vi "Launch Instruments.vi"(8 "error in":errorcluster, 11 "Controller in":refnum<class "Controller.lvclass">) -> (0 "error out":errorcluster, 3 "Controller out":refnum<class "Controller.lvclass">)   [LabVIEW 2018, in "Controller.lvlib" / "Controller.lvclass"]
doc: "Configure the Instrument objects for operation and stuff them in their appropriate Instr Actor objects, calling their Pre Launch Init methods. The queues for these will be stored in the FGV for communication with the UI."
uses:
  Controller.lvclass
  PAS/Instrument/ePAS.lvclass
  C:/Users/Labview/Documents/exscalabar_server/reusable/Instrument/Instrument.lvclass
  CRDS/Main/eCRDS.lvclass
  reusable/PAS/Data/Main/PAS Data.lvclass
  C:/Users/Labview/Documents/exscalabar_server/reusable/Data/Data.lvclass
  Instr Actor/Instr Actor.lvclass
  C:/Users/Labview/Documents/exscalabar_server/SuperActor/SuperActor.lvclass
  C:/Program Files (x86)/National Instruments/LabVIEW 2018/vi.lib/ActorFramework/Actor/Actor.lvclass
  PAS/Data/Cell/ePAS Cell Data.lvclass
  C:/Users/Labview/Documents/exscalabar_server/reusable/PAS/Data/Cell/PAS Cell Data.lvclass
  Update Controller Data MSG.lvclass
  C:/Users/Labview/Documents/exscalabar_server/reusable/DAQ Device/Device/Generic Data Update Data MSG/Generic Update Data Message.lvclass
  reusable/Instrument/Instrument.lvclass/Instrument.ctl
  reusable/DAQ Device/Device/Generic Data Update Data MSG/Generic Update Data Message.lvclass/Generic Update Data Message.ctl
  Instr Actor/Instr Actor.lvclass/Instr Actor.ctl
  SuperActor/SuperActor.lvclass/SuperActor.ctl
  reusable/DAQ Device/Device/Generic Data Update Data MSG/Write ID.vi
  Instr Actor/Accessors/Write Instr.vi
  SuperActor/Write ID.vi
  Instr Actor/Accessors/Write Update Data MSG.vi
  reusable/Instrument/Write Data.vi
  reusable/PAS/Data/Main/Write CellData.vi
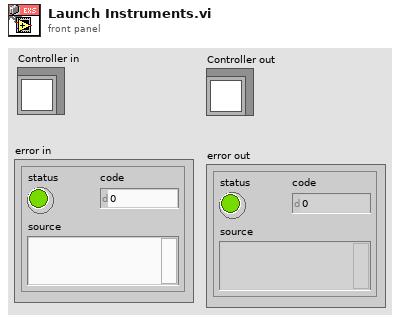
[diagram p1: front panel]
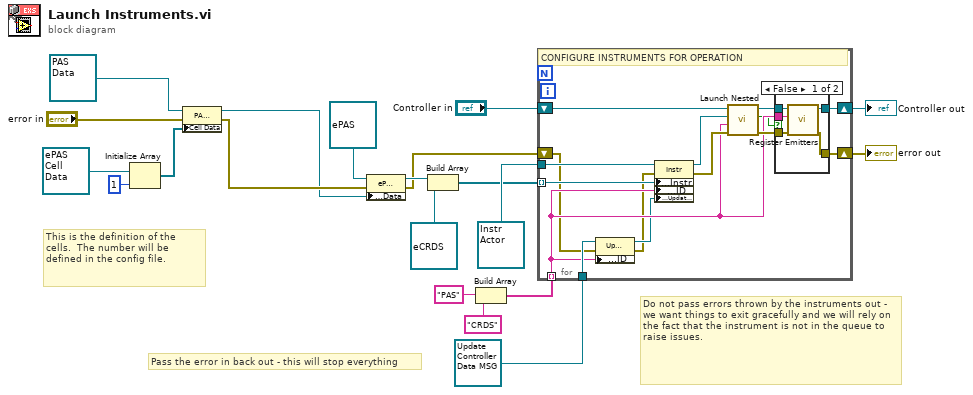
[diagram p0: block diagram]
diagram:
  # "This is the definition of the cells.  The number will be defined in the config file."
  # "Do not pass errors thrown by the instruments out - we want things to exit gracefully and we will rely on the fact that the instrument is not in the queue to raise issues."
  # "Pass the error in back out - this will stop everything"
  n1 = Initialize Array(refnum<class "ePAS Cell Data.lvclass"> refnum ("ePAS Cell"), 1 ("dimension size")) -> (w17:refnum<class "ePAS Cell Data.lvclass">[])
  n2 = property class="PAS Data"(reference=refnum<class "PAS Data.lvclass"> refnum ("PAS Data"), error in="error in", "Cell Data"=w17) -> (reference out=w11:refnum<class "PAS Data.lvclass">, error out=w18:errorcluster)
  n3 = property class="ePAS"(reference=refnum<class "ePAS.lvclass"> refnum ("ePAS.lvclass"), error in=w18, "Accessors:Data"=w11) -> (reference out=w15:refnum<class "ePAS.lvclass">, error out=w9:errorcluster)
  n4 = Build Array(w15, refnum<class "eCRDS.lvclass"> refnum ("eCRDS")) -> (w12:refnum<class "Instrument.lvclass">[])
  n5 = Build Array("PAS", "CRDS" ("element")) -> (w6:string[])
  n6 = for {
    tunnel: w12 -> [w35] mode=indexing
    tunnel: refnum<class "Instr Actor.lvclass"> refnum ("Instrument Lib:Instr") -> [w34]
    tunnel: w6 -> [w25] mode=indexing
    shift-right: [w28] -> w4
    shift-left: "Controller in" -> [w33]
    shift-right: [w27] -> w2
    shift-left: w9 -> [w23]
    tunnel: refnum<class "Update Controller Data MSG.lvclass"> refnum ("Controller.lvlib:Update Data MSG") -> [w26]
    # "CONFIGURE INSTRUMENTS FOR OPERATION"
    n7 = property class="Update Data MSG"(reference=w26, error in=w23, "Accessors:ID"=w25) -> (reference out=w24:refnum<class "Update Controller Data MSG.lvclass">, error out=w22:errorcluster)
    n8 = property class="Instr"(reference=w34, error in=w22, "Accessors:Instr"=w35, "Accessors:ID"=w25, "Accessors:Update Data MSG"=w24) -> (reference out=w32:refnum<class "Instr Actor.lvclass">, error out=w31:errorcluster)
    n9 = call "Launch Nested.vi"("Error In"=w31, "ID"=w25, "Nested Actor"=w32, "Controller in"=w33) -> ("Error Out"=w29:errorcluster, "Launch Failure?"=w21:bool, "Controller out"=w30:refnum<class "Controller.lvclass">)  [unwired: 4 in, 1 out]
    n10 = case shown="False" w21 {
      tunnel: w30 -> [w40 w42]
      tunnel: w29 -> [w39 w41]
      tunnel: [w38 w42] -> w28
      tunnel: [w37 w41] -> w27
      tunnel: w25 -> [w36 _]
      frame False {
        n11 = call "Register Emitters.vi"("error in"=w39, "Emitter"=w36, "Controller in"=w40) -> ("error out"=w37:errorcluster, "Controller out"=w38:refnum<class "Controller.lvclass">)  [unwired: 7 in]
      }
      frame True {
      }
    }
  }
  "Controller out" <- w4
  "error out" <- w2
